vi "Set Attribute Tree Data.vi"(7 "Tree ID":string, 8 "Error In":errorcluster, 9 "Attribute Value":refnum<class "Tree Data.lvclass">, 10 "Attribute Name":string, 11 "Tree Manager":T1) -> (0 "Error Out":errorcluster, 1 "Replaced?":bool, 3 "Tree Manager":T1)   [LabVIEW 2020, in "NI_VIAnCFGDataStructure.lvlib" / "Tree.lvclass"]
doc: "Set a Tree Data object as an attribute of the Tree."
uses:
  <vilib>/addons/analyzer/VIAnCFGDataStructure/Tree Manager/Tree.lvclass
  <vilib>/addons/analyzer/VIAnCFGDataStructure/Tree Manager/Typedefs/Session Handle.ctl
  <vilib>/addons/analyzer/VIAnCFGDataStructure/Tree Data/Tree Data.lvclass
  <vilib>/addons/analyzer/VIAnCFGDataStructure/Tree Manager/Tree.lvclass/Tree.ctl
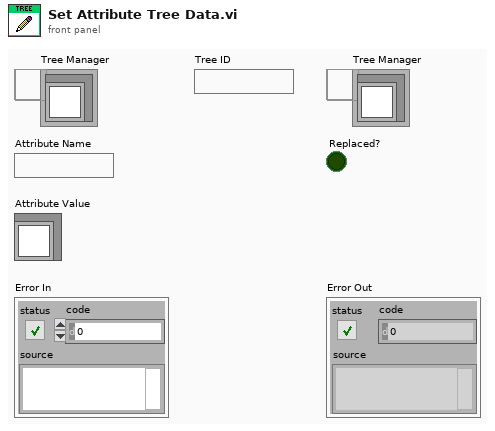
[diagram p1: front panel]
types:
  T1 = typedef "NI_VIAnCFGDataStructure.lvlib/Tree.lvclass/Session Handle.ctl" = refnum<data-value>
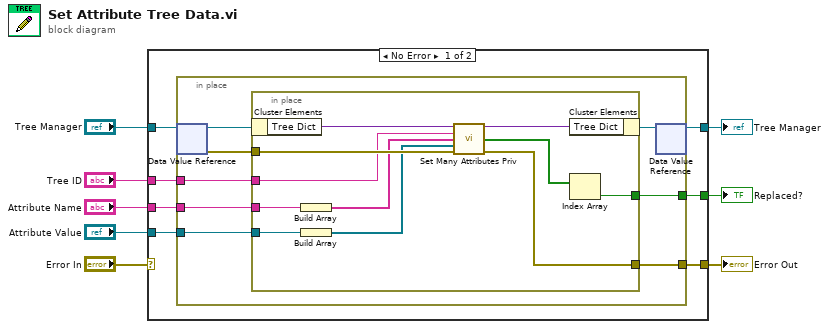
[diagram p0: block diagram]
diagram:
  n1 = case shown="No Error" "Error In" {
    selector: "Error In" -> [_ w35]
    tunnel: "Tree Manager" -> [w15 w36]
    tunnel: [w14 w36] -> w7
    tunnel: [w13 w35] -> w5
    tunnel: "Tree ID" -> [w12 _]
    tunnel: "Attribute Value" -> [w11 _]
    tunnel: "Attribute Name" -> [w10 _]
    tunnel: [w9 _] -> w2
    frame No Error {
      n2 = in-place {
        in-place-border: [w20] -> w13
        in-place-border: w12 -> [w16]
        in-place-border: w11 -> [w19]
        in-place-border: w10 -> [w18]
        in-place-border: [w21] -> w9
        n3 = in-place-dvr #1(w15) -> (w23:refnum<class "Tree.lvclass">, w17:errorcluster)
        n4 = in-place {
          in-place-border: [w26] -> w20
          in-place-border: w17 -> [w32]
          in-place-border: w16 -> [w27]
          in-place-border: w19 -> [w34]
          in-place-border: w18 -> [w33]
          in-place-border: [w24] -> w21
          n5 = in-place-cluster #2(w23) -> ("Tree Dict"=w31:variant)
          n6 = Build Array(w33) -> (w28:string[])
          n7 = Build Array(w34) -> (w29:refnum<class "Tree Data.lvclass">[])
          n8 = call <vilib>:"Set Many Attributes Priv.vi"("Tree Dictionary Out"=w31, "Unique ID"=w27, "Name"=w28, "Data"=w29, "error in"=w32) -> ("Tree Dictionary Out"=w30:variant, "Replaced?"=w25:bool[], "error out"=w26:errorcluster)  [unwired: 8 in]
          n9 = in-place-cluster #2("Tree Dict"=w30) -> (w22:refnum<class "Tree.lvclass">)
          n10 = Index Array(array=w25) -> (element=w24:bool)  [unwired: 1 in]
        }
        n11 = in-place-dvr #1(w22) -> (w14:T1)  [unwired: 1 out]
      }
    }
    frame Error {
    }
  }
  "Tree Manager" <- w7
  "Error Out" <- w5
  "Replaced?" <- w2
